vi "search4objINFO.vi"(7 "obj properties of interest":string[](array[string]), 8 "dxfObject in":T1, 10 "complete obj in":string[][](array[string])) -> (3 "obj of interest data out":string[](array[string]), 5 "dxfObject of interest out":T1)   [LabVIEW 2016, in "Dxf.lvlib"]
uses:
  Dxf.lvlib
  typeDefs/singleDXFobject.ctl
  typeDefs/singleDXFvar.ctl
  dxf typedef.lvlib
panel:
  # "Connector Pane"
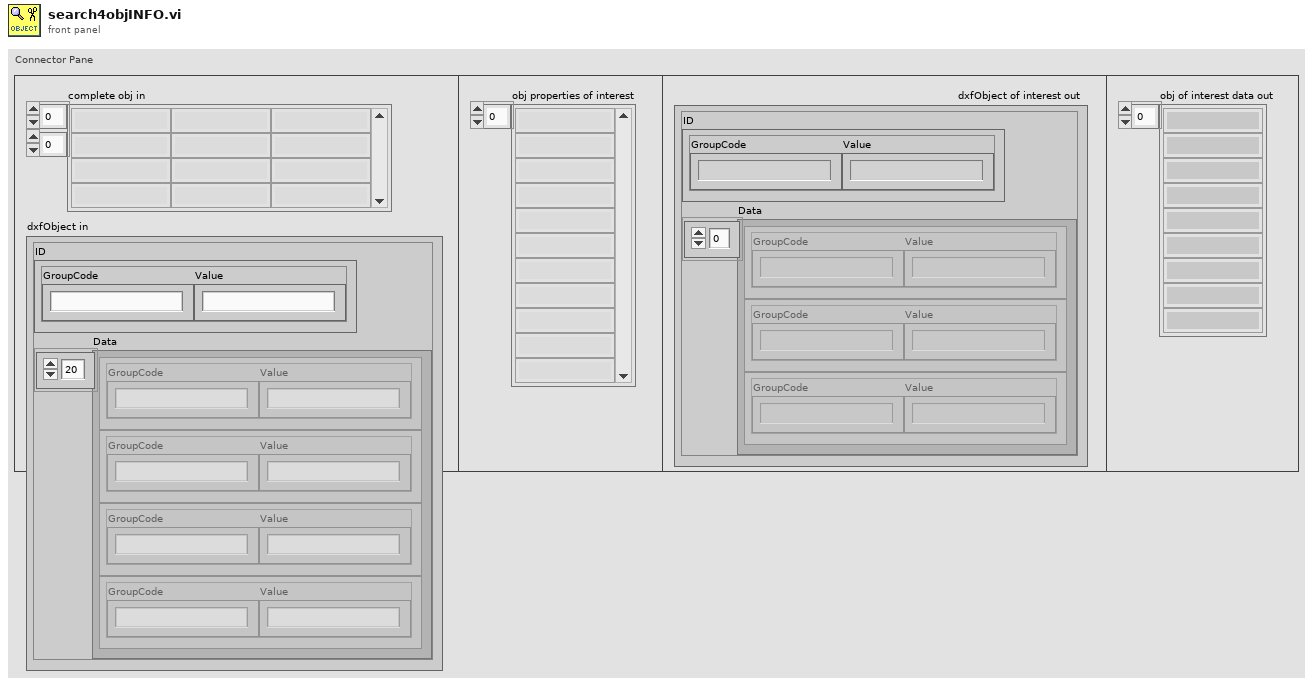
[diagram p1: front panel]
types:
  T1 = typedef "dxf typedef.lvlib/singleDXFobject.ctl" = cluster{"ID":T2, "Data":T2[]}
  T2 = typedef "dxf typedef.lvlib/singleDXFvar.ctl" = cluster{"GroupCode":string, "Value":string}
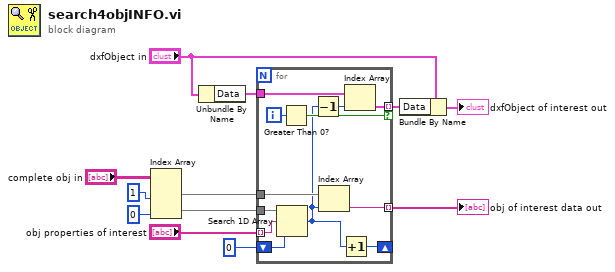
[diagram p0: block diagram]
diagram:
  n1 = Index Array(array="complete obj in", index (col) #1=1 ("disabled index (col)"), index (col) #2=0 ("disabled index (col)")) -> (element #1=w11:string[], element #2=w12:string[])  [unwired: 2 in]
  n2 = Unbundle By Name("dxfObject in") -> ("Data"=w5:T2[])
  n3 = for {
    tunnel: w12 -> [w24]
    tunnel: "obj properties of interest" -> [w23] mode=indexing
    tunnel: w11 -> [w22]
    tunnel: [w21] -> w9 mode=indexing
    tunnel: w5 -> [w20]
    tunnel: [w19] -> w4 mode=indexing if=w17
    shift-right: [w14] -> _
    shift-left: 0 ("disabled index (col)") -> [w15]
    i -> [w18]
    n4 = Search 1D Array(1D array=w24, element=w23, start index (0)=w15) -> (index of element=w13:i32)
    n5 = Greater Than 0?(x=w18) -> (x > 0?=w17:bool)
    n6 = Decrement(x=w13) -> (x-1=w16:i32)
    n7 = Index Array(array=w22, index=w13) -> (element=w21:string)
    n8 = Increment(x=w13) -> (x+1=w14:i32)
    n9 = Index Array(array=w20, index=w16) -> (element=w19:T2)
  }
  "obj of interest data out" <- w9
  n10 = Bundle By Name(cluster="dxfObject in", "Data"=w4) -> (→"dxfObject of interest out":T1)
